vi "生成监听数据.vi"(11 "监听数据":string[](array[string])=["时间", "操作", "数据(HEX)"]) -> (3 "输出数组":string[][](array[string]))   [LabVIEW 2015]
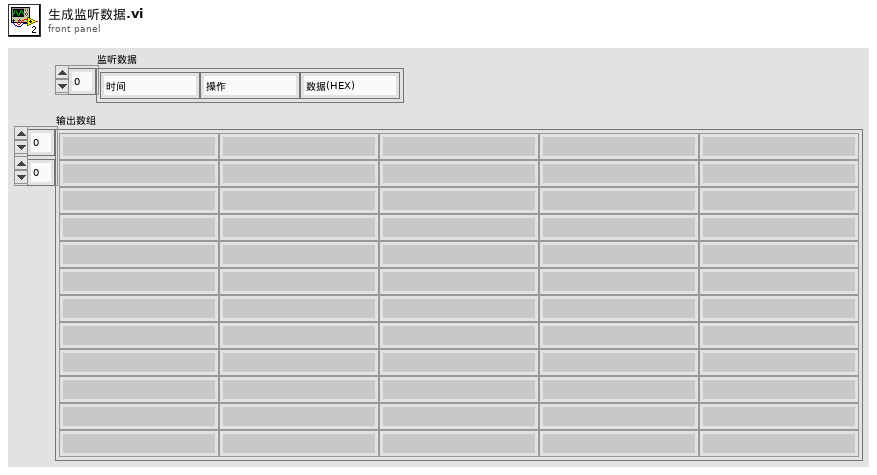
[diagram p1: front panel]
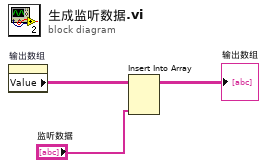
[diagram p0: block diagram]
diagram:
  n1 = property on="输出数组" class="Arr (严格)"() -> ("Value"=w2:string[][])  [unwired: 2 in, 2 out]
  n2 = Insert Into Array(array=w2, new element="监听数据") -> (→"输出数组":string[][])  [unwired: 2 in]
